vi "ReadTracepoints.vi"(8 "error in (no error)":errorcluster, 11 "log dir":path) -> (0 "error out":errorcluster)   [LabVIEW 2017, in "TraceLogger.lvlib"]
uses:
  <vilib>/addons/TraceLogger/TraceLogger.lvlib
  <vilib>/addons/TraceLogger/controls/TracepointConfig.ctl
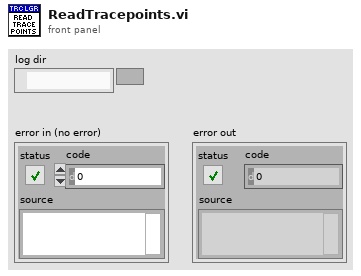
[diagram p1: front panel]
types:
  T1 = typedef "TraceLogger.lvlib/TracepointConfig.ctl" = cluster{"name":string, "enabled":bool}
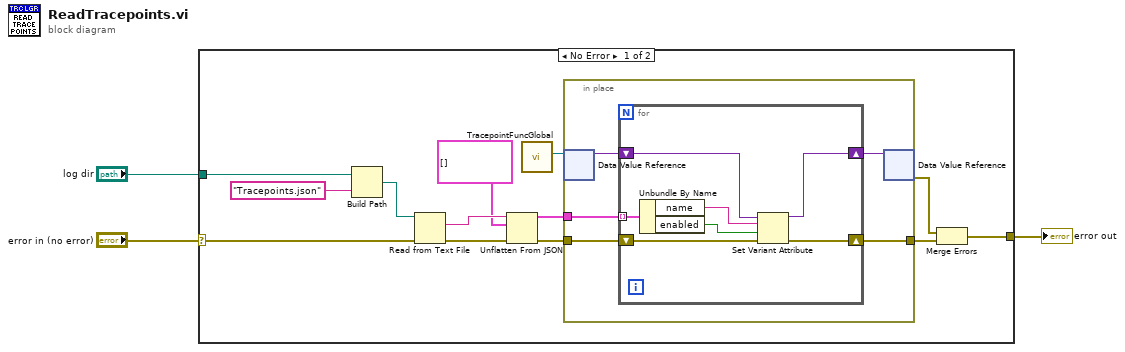
[diagram p0: block diagram]
diagram:
  n1 = case shown="No Error" "error in (no error)" {
    selector: "error in (no error)" -> [w9 w29]
    tunnel: [w5 w29] -> w3
    tunnel: "log dir" -> [w8 _]
    frame No Error {
      n2 = Build Path(base path=w8, name or relative path="Tracepoints.json") -> (appended path=w15:path)
      n3 = Read from Text File(file (use dialog)=w15, error in=w9) -> (text=w13:string, error out=w14:errorcluster)  [unwired: 2 in, 2 out]
      n4 = Unflatten From JSON(JSON string=w13, type and defaults=T1[] [], error in (no error)=w14) -> (value=w11:T1[], error out=w10:errorcluster)  [unwired: 4 in]
      n5 = call <vilib>:"TracepointFuncGlobal.vi"() -> ("tracepoints"=w7:refnum<data-value>)  [unwired: 11 in]
      n6 = in-place {
        in-place-border: w11 -> [w21]
        in-place-border: w10 -> [w20]
        in-place-border: [w19] -> w4
        n7 = in-place-dvr #1(w7) -> (w18:variant)  [unwired: 1 out]
        n8 = for {
          tunnel: w21 -> [w26] mode=indexing
          shift-right: [w28] -> w17
          shift-left: w18 -> [w27]
          shift-right: [w24] -> w19
          shift-left: w20 -> [w23]
          n9 = Unbundle By Name(w26) -> ("name"=w25:string, "enabled"=w22:bool)
          n10 = Set Variant Attribute(Variant=w27, name=w25, value=w22, error in=w23) -> (Variant out=w28:variant, error out=w24:errorcluster)  [unwired: 1 out]
        }
        n11 = in-place-dvr #1(w17) -> (w6:errorcluster)  [unwired: 1 out]
      }
      n12 = Merge Errors(w6, w4) -> (w5:errorcluster)
    }
    frame Error {
    }
  }
  "error out" <- w3
